vi "Is Conainer Frozen.vi"(6 "Frozen threshold (-160C)":dbl=-160.0, 7 "Container":T1, 8 "error in (no error)":errorcluster, 11 "cRIO-CO2 in":refnum<class "cRIO-CO2.lvclass">) -> (0 "error out":errorcluster, 1 "Is Frozen?":bool, 2 "Temperature":dbl, 3 "cRIO-CO2 out":refnum<class "cRIO-CO2.lvclass">)   [LabVIEW 2015, in "cRIO-Carbondioxide.lvlib" / "cRIO-CO2.lvlib" / "cRIO-CO2.lvclass"]
uses:
  cRIO-CO2.lvclass
  Controls/Sample Transfer Container Enumerator.ctl
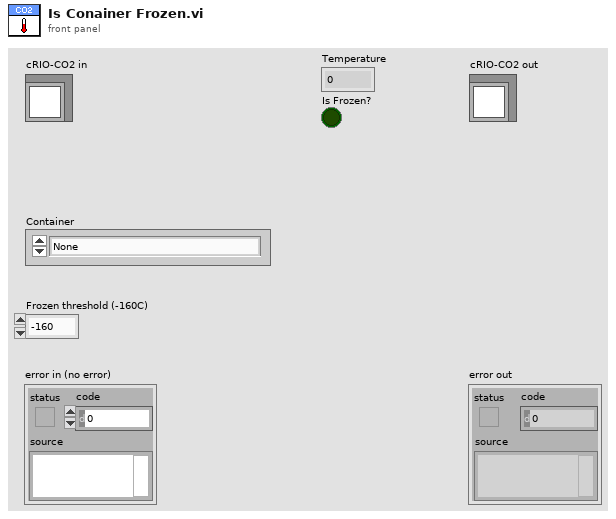
[diagram p1: front panel]
types:
  T1 = typedef "Sample Transfer Container Enumerator.ctl" = enum16{"None", "Sample 1", "Sample 2", "Sample 3", "Sample 4", "Sample 5", "Storage 01", "Storage 02", "Storage 03", "Storage 04", "Storage 05", "Storage 06", "Storage 07", "Storage 08", "Storage 09", "Storage 10", "Storage 11", "Storage 12", "Syringe", "Undefined"}
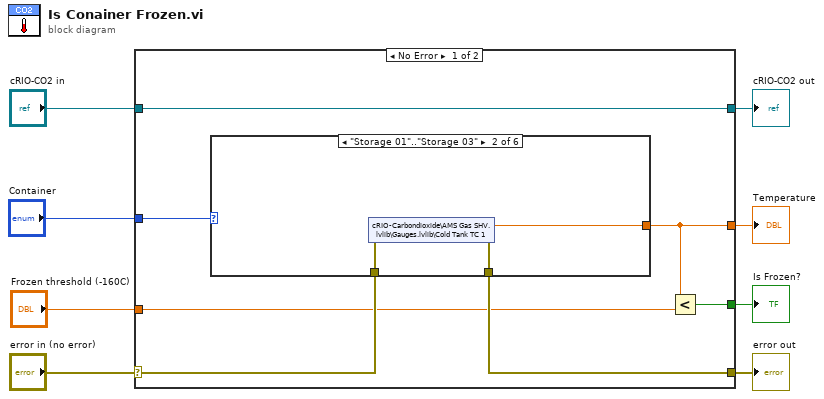
[diagram p0: block diagram]
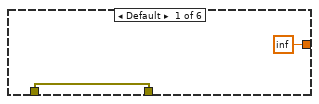
[diagram p2: hidden frame]
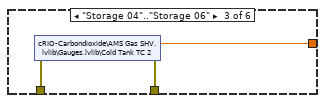
[diagram p3: hidden frame]
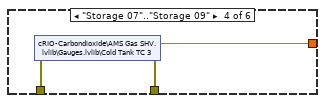
[diagram p4: hidden frame]
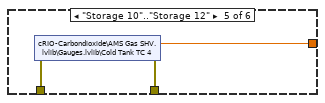
[diagram p5: hidden frame]
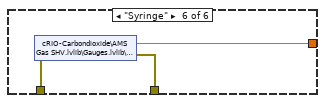
[diagram p6: hidden frame]
diagram:
  n1 = case shown="No Error" "error in (no error)" {
    selector: "error in (no error)" -> [w13 w34]
    tunnel: [w12 w34] -> w7
    tunnel: [w15 w33] -> w5
    tunnel: "cRIO-CO2 in" -> [w15 w33]
    tunnel: "Container" -> [w14 _]
    tunnel: [w10 _] -> w3
    tunnel: "Frozen threshold (-160C)" -> [w11 _]
    tunnel: [w9 _] -> w1
    frame No Error {
      n2 = case shown="\"Storage 01\"..\"Storage 03\"" w14 {
        tunnel: w13 -> [w16 w20 w23 w26 w29 w32]
        tunnel: [w16 w19 w22 w25 w28 w30] -> w12
        tunnel: [inf ("Double") w18 w21 w24 w27 w31] -> w10
        frame Default {
        }
        frame "Storage 01".."Storage 03" {
          n3 = shared-variable "cRIO-Carbondioxide\\AMS Gas SHV.lvlib\\Gauges.lvlib\\Cold Tank TC 1"(error in=w20) -> (w18:dbl, error out=w19:errorcluster)
        }
        frame "Storage 04".."Storage 06" {
          n4 = shared-variable "cRIO-Carbondioxide\\AMS Gas SHV.lvlib\\Gauges.lvlib\\Cold Tank TC 2"(error in=w23) -> (w21:dbl, error out=w22:errorcluster)
        }
        frame "Storage 07".."Storage 09" {
          n5 = shared-variable "cRIO-Carbondioxide\\AMS Gas SHV.lvlib\\Gauges.lvlib\\Cold Tank TC 3"(error in=w26) -> (w24:dbl, error out=w25:errorcluster)
        }
        frame "Storage 10".."Storage 12" {
          n6 = shared-variable "cRIO-Carbondioxide\\AMS Gas SHV.lvlib\\Gauges.lvlib\\Cold Tank TC 4"(error in=w29) -> (w27:dbl, error out=w28:errorcluster)
        }
        frame "Syringe" {
          n7 = shared-variable "cRIO-Carbondioxide\\AMS Gas SHV.lvlib\\Gauges.lvlib\\Syringe TC"(error in=w32) -> (w31:dbl, error out=w30:errorcluster)
        }
      }
      n8 = Less?(x=w10, y=w11) -> (x < y?=w9:bool)
    }
    frame Error {
    }
  }
  "error out" <- w7
  "cRIO-CO2 out" <- w5
  "Temperature" <- w3
  "Is Frozen?" <- w1
